vi "Constants.vi"() -> ()   [LabVIEW 2017, in "ALMA_10201-10401_O2SensorSim Shared.lvlib"]
doc: "Use this Global VI to access the GUIDs assigned to the page resources of the Custom Device."
uses:
  ALMA_10201-10401_O2SensorSim Shared.lvlib
panel:
  in  "Tab Control":enum32{"GUIDS", "Constants", "Properties"}(tab)
  in  "PID Ch":string="c82b20b8-f784-4ce0-9686-ded74c652b67"
  in  "Feedback Ch":string="c82b20b8-f784-4ce0-9686-ded74c652b66"
  in  "Setpoint Ch":string="c82b20b8-f784-4ce0-9686-ded74c652b65"
  in  "Status Ch":string="c82b20b8-f784-4ce0-9686-ded74c652b64"
  in  "PID":string="5eaf23de-b745-4c98-9863-0727b1949209"
  in  "Feedback":string="5eaf23de-b745-4c98-9863-0727b1949208"
  in  "Setpoint":string="5eaf23de-b745-4c98-9863-0727b1949207"
  in  "Status":string="5eaf23de-b745-4c98-9863-0727b1949206"
  in  "GUID EnableDisable Page":string="ec94fc63-336f-4d75-8121-0362e05bb837"
  in  "Page2":string="1a22a596-5480-47c7-a053-b94d1eca3b0e"
  in  "Page1":string="e034f56b-6ead-4a7d-959d-73e50ffe2abf"
  in  "O2SensorSim_SLSC":string="b95ed1a2-440b-4256-b4a3-412d4d53b190"
  in  "product.Num_4ch":i32=10401
  in  "Module.Name_4ch":string="SLSC-Alma 4CH O2 Simul Module"
  in  "CD Version":string="1.0.0"
  in  "vendor.Num":i32=4141
  in  "product.Num_2ch":i32=10201
  in  "Module.Name_2ch":string="SLSC-Alma 2CH O2 Simul Module"
  in  "Channel Interface Name":string="Channel Interface"
  in  "CHM File Name":string="SLSC Module Addon.chm"
  in  "Caps Version":string="1.0.0"
  in  "Documentation":string="Documentation"
  in  "initialized?":string="initialized"
  in  "Chassis IP Address":string="Chassis IP Address"
  in  "Chassis #":string="Chassis #"
  in  "Module Number":string="Slot #"
  in  "ModuleName":string="ModuleName"
  in  "SLSC Plug-in Names":string="SLSC Plug-in Names"
  in  "SLSC Plug-in GUIDs":string="SLSC Plug-in GUIDs"
  in  "SLSC Plug-in Paths":string="SLSC Plug-in Paths"
  in  "SLSC Root CD Version":string="SLSC Root CD Version"
  in  "Slot CD Processor Affinity":string="Slot CD Processor Affinity"
  in  "vendorNum":string="vendorNum"
  in  "productNum":string="productNum"
  in  "Compiled.Settings":string="Compiled.Settings"
  in  "Page Configuration Settings":string="Page Configuration Settings"
  in  "PropertyNames":string="PropertyNames"
  in  "SLSCChannelPath":string="SLSCChannelPath"
  in  "Bank 0":string="Bank 0"
  in  "Output from SLSC":string="Output"
  in  "Status Channel":string="Diagnostics"
  in  "Command Channel":string="Commands"
  in  "Chassis Username":string="Chassis Username"
  in  "Input to SLSC":string="Input"
  in  "Bank 1":string="Bank 1"
  in  "capsVersion":string="capsVersion"
  in  "vendorNumber":string="vendorNumber"
  in  "productNumber":string="productNumber"
  in  "Revision A":string="RevA"
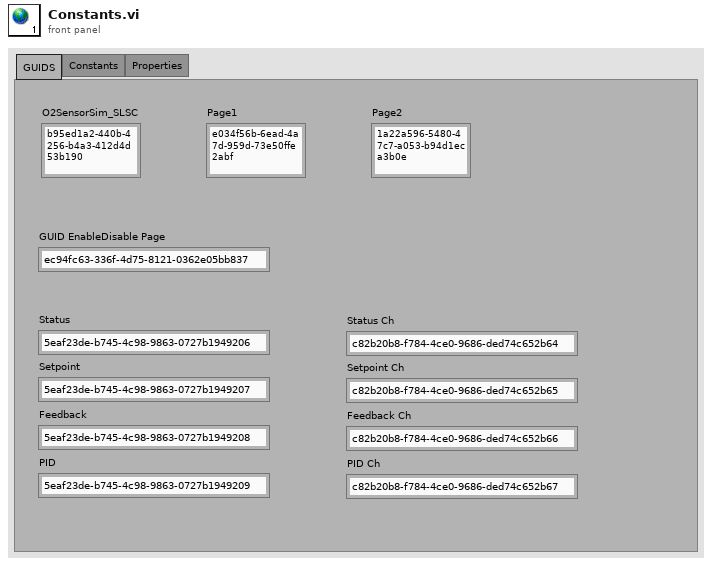
[diagram p1: front panel]
diagram:
